vi "RectToCoordinates.vi"(3 "Rect":T2) -> (1 "Coordinates":T1)   [LabVIEW 2014, in "WebFrontPanel.lvclass"]
uses:
  WebFrontPanel.lvclass
  <vilib>/Utility/miscctls.llb/LVRectTypeDef.ctl
  Object_class/Coordinates.ctl
  Object_class/Object.lvclass
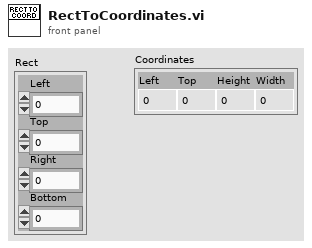
[diagram p1: front panel]
types:
  T1 = typedef "Object.lvclass/Coordinates.ctl" = cluster{"Left":i32, "Top":i32, "Height":u32, "Width":u32}
  T2 = typedef "LVRectTypeDef.ctl" = cluster{"Left":i16, "Top":i16, "Right":i16, "Bottom":i16}
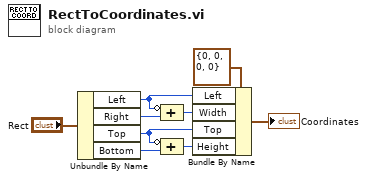
[diagram p0: block diagram]
diagram:
  n1 = Unbundle By Name("Rect") -> ("Left"=w6:i16, "Right"=w7:i16, "Top"=w3:i16, "Bottom"=w5:i16)
  n2 = Compound Arithmetic op=ADD(invert w6, w7) -> (w2:i16)
  n3 = Compound Arithmetic op=ADD(invert w3, w5) -> (w4:i16)
  n4 = Bundle By Name(cluster=T1 {"Left"=0, "Top"=0, "Height"=0, "Width"=0} ("Coordinates"), "Left"=w6, "Width"=w2, "Top"=w3, "Height"=w4) -> (→"Coordinates":T1)
